vi "Dioptriewert_setzen.vi"(8 "Fehler in":errorcluster, 10 "Dioptrie-Wert":dbl, 11 "Flüssiglinse in":refnum<k5>) -> (0 "Fehler out":errorcluster, 3 "Flüssiglinse out":refnum<k5>)   [LabVIEW 2024]
panel:
  out "Antwort Gardasoft":string
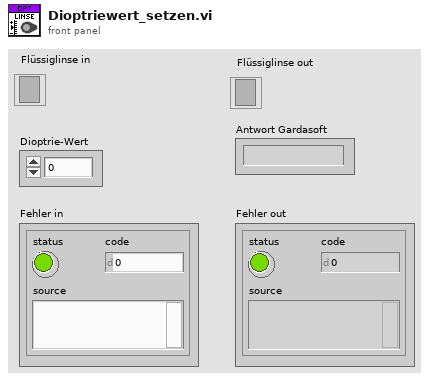
[diagram p1: front panel]
types:
  T1 = enum16{"Standard", "Buffered", "CRLF", "Immediate"}
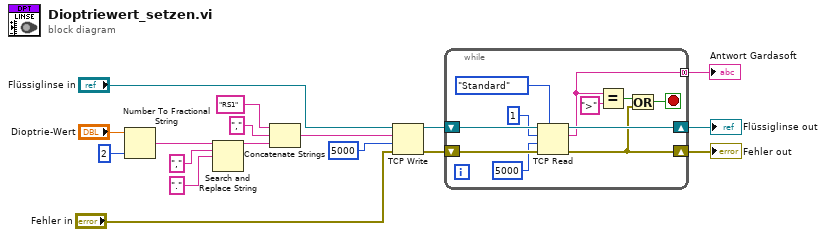
[diagram p0: block diagram]
diagram:
  n1 = Number To Fractional String(number="Dioptrie-Wert", precision (6)=i16 2 ("Genauigkeit (6)")) -> (F-format string=w16:string)  [unwired: 2 in]
  n2 = Search and Replace String(input string=w16, search string="," ("Such-String"), replace string="." ("Ersetzungs-String (\"\")")) -> (result string=w12:string)  [unwired: 5 in, 3 out]
  n3 = Concatenate Strings("RS1" ("String"), "," ("String"), w12) -> (w11:string)
  n4 = TCP Write(connection ID="Flüssiglinse in", data in=w11, error in (no error)="Fehler in", 9:5000 ("Timeout in ms (25000)")) -> (connection ID out=w8:refnum<k5>, error out=w7:errorcluster)  [unwired: 1 out]
  n5 = while {
    shift-right: [w26] -> w2
    shift-left: w8 -> [w28]
    shift-right: [w20] -> w3
    shift-left: w7 -> [w27]
    tunnel: [w18] -> w1 mode=concatenating
    stop <- w21 stop-if-true
    n6 = TCP Read(connection ID=w28, bytes to read=1 ("Zu lesende Bytes"), error in (no error)=w27, 7:T1."Standard" ("Modus (Standard)"), 9:5000 ("timeout ms (25000)")) -> (connection ID out=w26:refnum<k5>, data out=w18:string, error out=w20:errorcluster)
    n7 = Equal?(x=w18, y=">") -> (x = y?=w22:bool)
    n8 = Or(x=w22, y=w20) -> (x .or. y?=w21:bool)
  }
  "Fehler out" <- w3
  "Flüssiglinse out" <- w2
  "Antwort Gardasoft" <- w1
